vi "Initialize Configuration.vi"(8 "error in (no error)":errorcluster, 9 "settings":T1, 10 "name":string, 11 "Configuration in":refnum<class "Configuration.lvclass">) -> (0 "error out":errorcluster, 3 "Configuration out":refnum<class "Configuration.lvclass">)   [LabVIEW 2017, in "Data Sharing Framework Core.lvlib" / "Data Sharing Framework Engine.lvlib" / "Configuration.lvclass"]
uses:
  Configuration.lvclass
  Configuration/1.0.0/Public/Controls/DSF Settings Info.ctl
  Configuration.lvclass/Configuration.ctl
  Configuration/1.0.0/Data Sharing Framework Configuration.lvlib
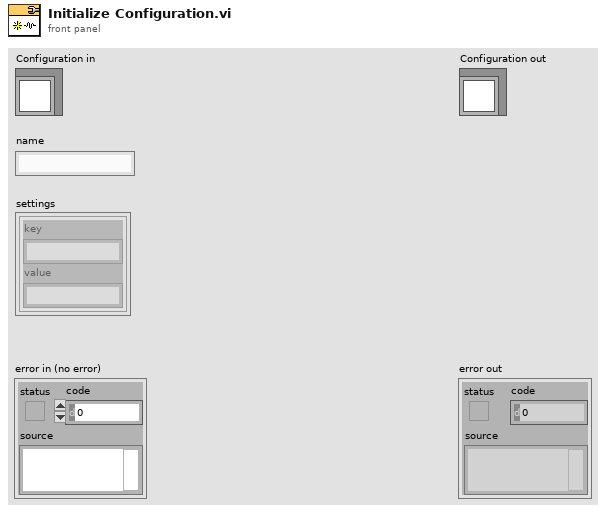
[diagram p1: front panel]
types:
  T1 = typedef "Data Sharing Framework Core.lvlib/Data Sharing Framework Configuration.lvlib/DSF Settings Info.ctl" = cluster{"key":string, "value":string}[]
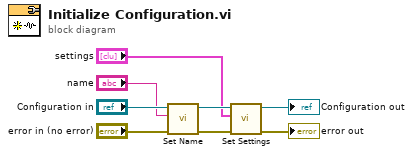
[diagram p0: block diagram]
diagram:
  n1 = call "Set Name.vi"("name"="name", "Configuration in"="Configuration in") -> ("Configuration out"=w5:refnum<class "Configuration.lvclass">)  [unwired: 9 in]
  n2 = call "Set Settings.vi"("settings"="settings", "Configuration in"=w5) -> ("Configuration out"=→"Configuration out":refnum<class "Configuration.lvclass">)  [unwired: 9 in]
  "error out" <- "error in (no error)"
